vi "P116x1ch_WriteAuto.vi"(7 "Decimales":u16(ring)=1 items=["0"=1, "1"=10, "2"=100], 8 "error in (no error)":errorcluster, 9 "RateSP(C/min)":T1, 10 "NuevoSP(C)":T1, 11 "Comunicaciones":T2={"Eurothe"="ASRL6::INSTR", "Eurot"=FALSE}) -> (0 "error out":errorcluster, 1 "NuevoRT2":T1, 2 "NuevoSP2":T1)   [LabVIEW 2017]
uses:
  1xP116.ctl
  Controles/P2024 COMMS.ctl
  Address.ctl
  Eurotherm_2023_Module.ctl
  P2024 Eurotherm GLOBALES.vi
panel:
  out "arrayRT":dbl[](array[numeric])
  out "arraySP":dbl[](array[numeric])
  out "PV":T1
  out "WorkingSP":T1
  out "TargetSP":T1
  in  "Cancel":bool
  in  "Write":bool
  out "Enable(T)":bool=TRUE
  out "VISA Promux":refnum<visa-resource-name>
  in  "Delay Time (s)":dbl=0.1
  # "Programando Eurotherm"
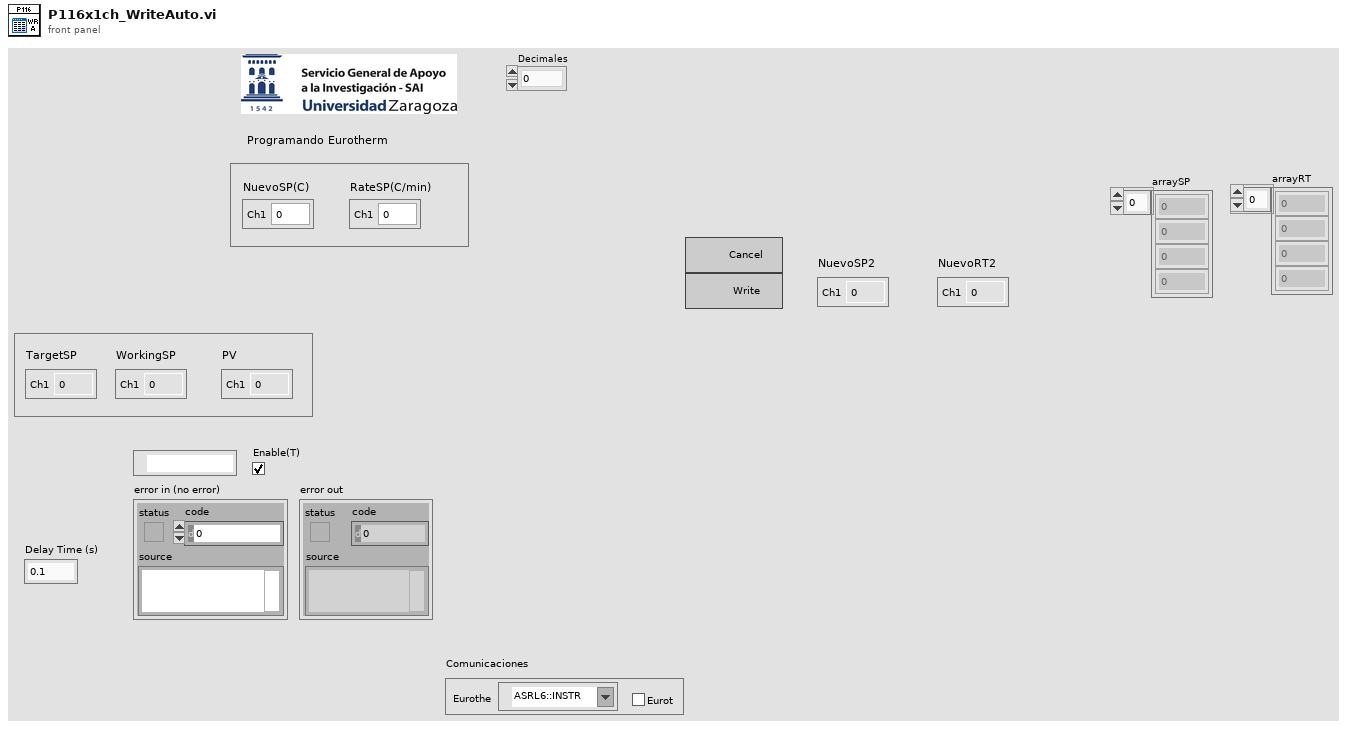
[diagram p1: front panel]
types:
  T1 = typedef "1xP116.ctl" = cluster{"Ch1":dbl}
  T2 = typedef "P2024 COMMS.ctl" = cluster{"Eurothe":refnum<visa-resource-name>, "Eurot":bool}
  T3 = typedef "P116x1ch.ctl" = cluster{"TargetSP":T1, "WorkingSP":T1, "Temperatura":T1, "RateSP":T1, "Potencia":T1, "Potencia max":T1}
  T4 = typedef "Eurotherm_2023_Module.ctl" = enum16{"Initialize", "Write setpoint", "Read data", "Write ramp rate", "Set constante proporcional", "Set constante integral", "Set constante diferencial", "Set ouput limit LOW", "Set ouput limit HIGH", "Shutdown"}
  T5 = typedef "Address.ctl" = enum16{"Add 1", "Add 2", "Add 3", "Add 4", "Add 5", "Add 6", "Add 10", "Add 11", "Add 12", "Add 13"}
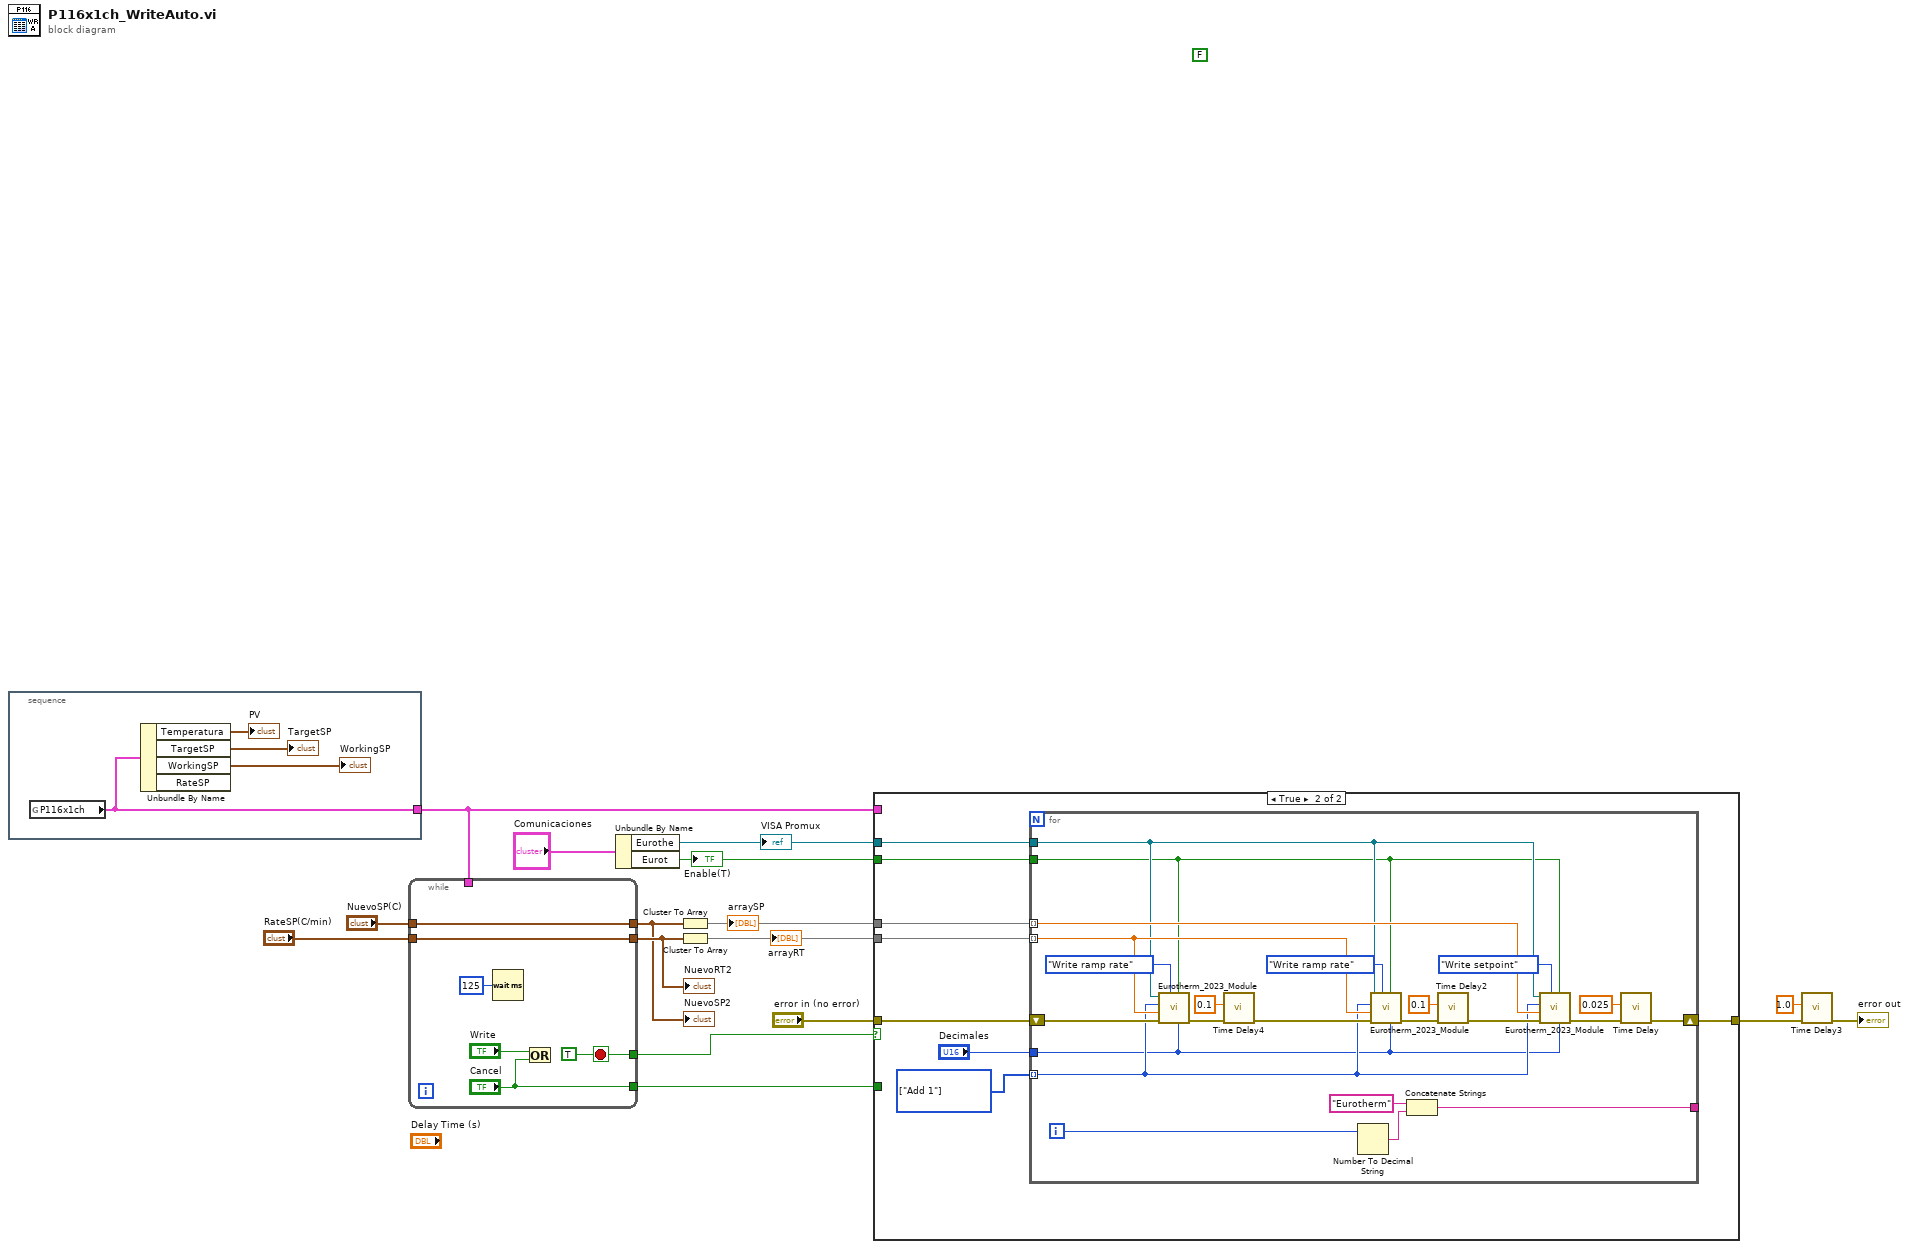
[diagram p0: block diagram]
diagram:
  (unwired) FALSE
  n1 = stacked-sequence {
    tunnel: [w17] -> w10
    frame #0 {
      n2 = global read "P2024 Eurotherm GLOBALES.vi" "P116x1ch"() -> (w17:T3)
      n3 = Unbundle By Name(w17) -> ("Temperatura"=→"PV":T1, "TargetSP"=→"TargetSP":T1, "WorkingSP"=→"WorkingSP":T1)  [unwired: 1 out]
    }
  }
  n4 = while {
    tunnel: ["Cancel"] -> w15
    tunnel: [w22] -> w8
    tunnel: [w23] -> w9
    tunnel: w10 -> [_]
    tunnel: "RateSP(C/min)" -> [w23]
    tunnel: "NuevoSP(C)" -> [w22]
    tunnel: [w21] -> w1
    stop <- w21 stop-if-true
    w21 = TRUE
    n5 = Wait (ms)(milliseconds to wait=u32 125) -> ()  [unwired: 1 out]
    n6 = Or(x="Write", y="Cancel") -> ()  [unwired: 1 out]
  }
  "NuevoSP2" <- w8
  "NuevoRT2" <- w9
  n7 = Unbundle By Name("Comunicaciones") -> ("Eurothe"=w11:refnum<visa-resource-name>, "Eurot"=w16:bool)
  "Enable(T)" <- w16
  "VISA Promux" <- w11
  n8 = Cluster To Array(cluster=w8) -> (array=w13:dbl[])
  "arraySP" <- w13
  n9 = Cluster To Array(cluster=w9) -> (array=w12:dbl[])
  "arrayRT" <- w12
  n10 = case shown="True" w1 {
    tunnel: w16 -> [_ w34]
    tunnel: w15 -> [_ _]
    tunnel: "error in (no error)" -> [w27 w33]
    tunnel: w13 -> [_ w31]
    tunnel: w12 -> [_ w32]
    tunnel: w11 -> [_ w35]
    tunnel: w10 -> [_ _]
    tunnel: [w27 w29] -> w5
    frame False {
    }
    frame True {
      w30 = T5[] [enum."Add 1"] items=["Add 1", "Add 2", "Add 3", "Add 4", "Add 5", "Add 6", "Add 10", "Add 11", "Add 12", "Add 13"]
      n11 = for {
        tunnel: w30 -> [w39] mode=indexing
        shift-right: [w49] -> w29
        shift-left: w33 -> [w53]
        tunnel: [w56] -> _
        tunnel: w31 -> [w51] mode=indexing
        tunnel: w32 -> [w40] mode=indexing
        tunnel: w35 -> [w38]
        tunnel: w34 -> [w37]
        tunnel: "Decimales" -> [w36]
        i -> [w48]
        n12 = call "Eurotherm_2023_Module.vi"("Decimales"=w36, "Eurotherm (T:Enable)"=w37, "Command"=Eurotherm_2023_Module."Write ramp rate", "error in (no error)"=w53, "Value"=w40, "Address"=w39, "VISA resource name"=w38) -> ("error out"=w42:errorcluster)  [unwired: 2 in, 2 out]
        n13 = call "Time Delay4"("error in (no error)"=w42, "Delay Time (s)"=0.1) -> ("error out"=w43:errorcluster)  [unwired: 9 in]
        n14 = Number To Decimal String(number=w48) -> (decimal integer string=w57:string)  [unwired: 1 in]
        n15 = call "Eurotherm_2023_Module.vi"("Decimales"=w36, "Eurotherm (T:Enable)"=w37, "Command"=Eurotherm_2023_Module."Write ramp rate", "error in (no error)"=w43, "Value"=w40, "Address"=w39, "VISA resource name"=w38) -> ("error out"=w41:errorcluster)  [unwired: 2 in, 2 out]
        n16 = Concatenate Strings("Eurotherm" ("error source (\" \")"), w57) -> (w56:string)
        n17 = call "Time Delay2"("error in (no error)"=w41, "Delay Time (s)"=0.1) -> ("error out"=w46:errorcluster)  [unwired: 9 in]
        n18 = call "Eurotherm_2023_Module.vi"("Decimales"=w36, "Eurotherm (T:Enable)"=w37, "Command"=Eurotherm_2023_Module."Write setpoint", "error in (no error)"=w46, "Value"=w51, "Address"=w39, "VISA resource name"=w38) -> ("error out"=w50:errorcluster)  [unwired: 2 in, 2 out]
        n19 = call "Time Delay"("error in (no error)"=w50, "Delay Time (s)"=0.025) -> ("error out"=w49:errorcluster)  [unwired: 9 in]
      }
    }
  }
  n20 = call "Time Delay3"("error in (no error)"=w5, "Delay Time (s)"=1.0) -> ("error out"=→"error out":errorcluster)  [unwired: 9 in]
